vi "Calculate Pump Power.vi"(1 "Motor temperature 2":u8, 2 "Motor temperature":u8, 3 "Acceleration pedal":dbl) -> (0 "Pumps power":dbl(slide) scale=0.0..100.0 scale format="%#_g%%")   [LabVIEW 2016]
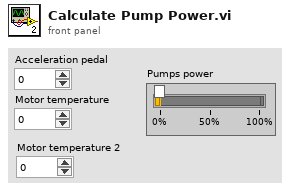
[diagram p1: front panel]
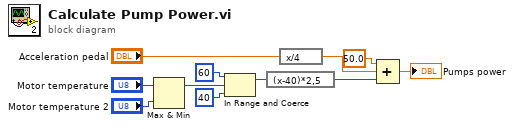
[diagram p0: block diagram]
diagram:
  n1 = Max & Min(x="Motor temperature", y="Motor temperature 2") -> (max(x,y)=w11:u8)  [unwired: 1 out]
  n2 = In Range and Coerce(upper limit=u8 60, x=w11, lower limit=u8 40) -> (coerced(x)=w8:u8)  [unwired: 1 out]
  n3 = expression code="(x-40)*2,5"(w8) -> (w6:u8)
  n4 = expression code="x/4"("Acceleration pedal") -> (w7:dbl)
  n5 = Compound Arithmetic op=ADD(50.0 ("value"), w7, w6) -> (→"Pumps power":dbl)
